vi "Close.vi.LOCAL.vi"(8 "error in (no error)":errorcluster, 11 "Masterflex Settings in":T1={"VISA resource name"="", "Simulated?"=FALSE, "Pump Number"=1.0, "Reverse?"=FALSE} {"Pump Number" min=1.0 max=20.0 step=1.0}) -> (0 "error out":errorcluster, 3 "Masterflex Settings out":T1={"VISA resource name"="", "Simulated?"=FALSE, "Pump Number"=1.0, "Reverse?"=FALSE} {"Pump Number" min=1.0 max=20.0 step=1.0})   [LabVIEW 2021, in "Masterflex 7550-30.lvlib"]
uses:
  Masterflex 7550-30.lvlib
  Controls/Settings Cluster.ctl
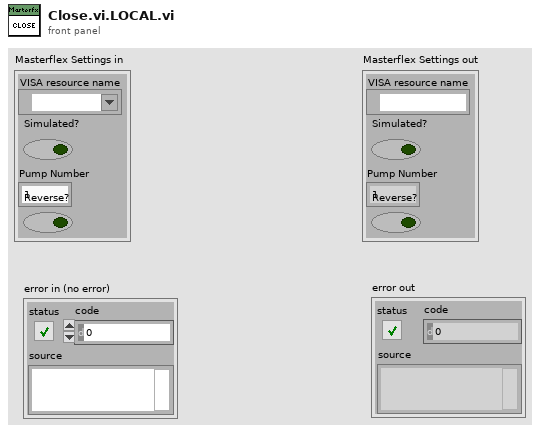
[diagram p1: front panel]
types:
  T1 = typedef "Masterflex 7550-30.lvlib/Settings Cluster.ctl" = cluster{"VISA resource name":refnum<visa-resource-name>, "Simulated?":bool, "Pump Number":dbl, "Reverse?":bool}
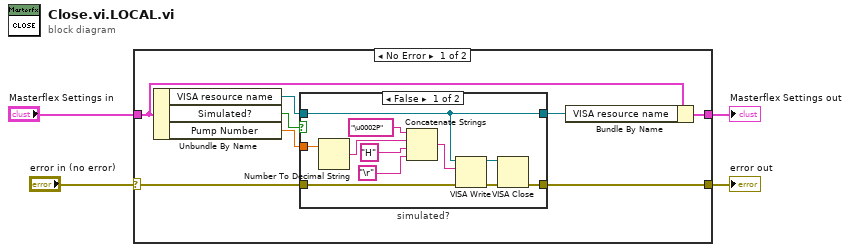
[diagram p0: block diagram]
diagram:
  n1 = case shown="No Error" "error in (no error)" {
    selector: "error in (no error)" -> [w11 w27]
    tunnel: [w10 w27] -> w4
    tunnel: [w9 w26] -> w1
    tunnel: "Masterflex Settings in" -> [w8 w26]
    frame No Error {
      n2 = Unbundle By Name(w8) -> ("VISA resource name"=w6:refnum<visa-resource-name>, "Simulated?"=w12:bool, "Pump Number"=w5:dbl)
      n3 = case "simulated?" shown="False" w12 {
        tunnel: [w23 w25] -> w10
        tunnel: w11 -> [w16 w25]
        tunnel: [w19 w24] -> w7
        tunnel: w6 -> [w19 w24]
        tunnel: w5 -> [w14 _]
        frame False {
          n4 = Number To Decimal String(number=w14) -> (decimal integer string=w13:string)  [unwired: 1 in]
          n5 = Concatenate Strings("\u0002P" ("string"), w13, "H" ("string"), "\r") -> (w15:string)
          n6 = VISA Write(VISA resource name=w19, write buffer=w15, error in (no error)=w16) -> (VISA resource name out=w18:refnum<visa-resource-name>, error out=w17:errorcluster)  [unwired: 1 out]
          n7 = VISA Close(VISA resource name=w18, error in (no error)=w17) -> (error out=w23:errorcluster)
        }
        frame True {
        }
      }
      n8 = Bundle By Name(cluster=w8, "VISA resource name"=w7) -> (w9:T1)
    }
    frame Error {
    }
  }
  "error out" <- w4
  "Masterflex Settings out" <- w1
